vi "Measurement UI.vi"() -> ()   [LabVIEW 2021, in "audio_adc_acDualChannelMeasurementUI.lvlib"]
uses:
  audio_adc_acDualChannelMeasurementUI.lvlib
  sub-vis/View.ctl
  sub-vis/Selector.ctl
  audio_adc_acDualChannelMeasurement.lvlib
panel:
  in  "MeasGraphs":T1(tab)
  in  "freq view":T2
  out "FreqDomainGraph":cluster{"x0":dbl, "dx":dbl, "magnitude":dbl[]}[](graph) caption="AC"
  in  "time view":T2
  out "TimeDomainGraph":waveform(dbl)[](graph) caption="AC"
  in  "Bit clock edge sync":u32=1
  in  "Frame sync pulse width":u32=32
  in  "Frame length":u32=64
  in  "Data justification":u32 caption="Data Justification"
  in  "Endianness":u32
  in  "Channel 0 offset":u32=1
  in  "Bit depth":u32=24
  in  "Channel length":u32=32
  in  "Channel count per frame":u32=2
  in  "Frame sync edge for channel 0":u32=1
  out "Spectrum":dbl[](array[numeric])
  out "df":dbl[](array[numeric])
  out "f0":dbl[](array[numeric])
  out "Time domain":dbl[](array[numeric])
  out "dt":dbl[](array[numeric])
  out "THD+N":dbl[](array[numeric])
  out "THD":dbl[](array[numeric])
  out "SNR":dbl[](array[numeric])
  out "Calculated amplitude":dbl[](array[numeric])
  out "Calculated frequency":dbl[](array[numeric])
  out "SFDR":dbl[](array[numeric])
  out "Dynamic range":dbl[](array[numeric])
  out "Gain error":dbl[](array[numeric])
  out "MeasTable":string[][](table)
  in  "Select":T3
  in  "Resource List":i32[](listbox)
  in  "Analog source resource name":string caption="RESOURCE NAME"
  in  "Configure Protocol Settings":bool
  in  "Protocol capture resource name":string(combo) caption="RESOURCE NAME"
  in  "Channel":string caption="CHANNEL"
  in  "Data line":u16 caption="DATA LINE"
  in  "Protocol settings":string="Protocol settings"
  in  "Analog source":string="Analog source "
  in  "Full scale range":dbl=2.825 caption="FULL SCALE RANGE" format="%.3pV"
  in  "Measurement settings":string="Measurement settings"
  in  "MeasSettingsOptions":i32(listbox)=-1
  in  "MeasSettings":bool
  in  "Weighting filter":string(combo)="Linear" caption="WEIGHTING FILTER"
  in  "Measurement duration":dbl=0.1 caption="MEASUREMENT DURATION" format="%#_6ps"
  in  "Sample rate":dbl=44100.0 caption="SAMPLE RATE" format="%#.6pHz"
  in  "Band stop":dbl=20000.0 caption="BAND STOP" format="%#_6pHz"
  in  "Band start":dbl=20.0 caption="BAND START" format="%#_6pHz"
  in  "Amplitude":dbl=-1.0 caption="AMPLITUDE" format="%#_6pdB"
  in  "Frequency":dbl=1000.0 caption="FREQUENCY" format="%#_6pHz"
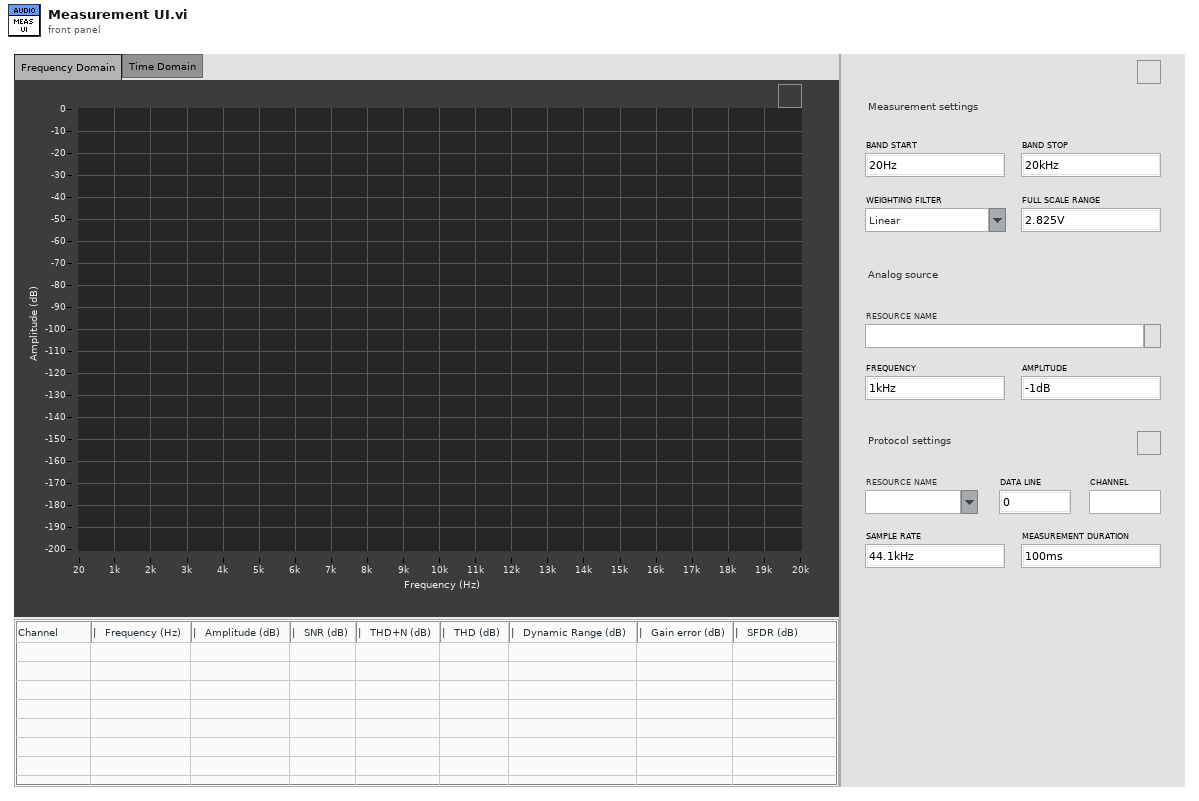
[diagram p1: front panel]
types:
  T1 = enum32{"Frequency Domain", "Time Domain", "Hidden Controls"}
  T2 = typedef "audio_adc_acDualChannelMeasurement.lvlib/View.ctl" = bool
  T3 = typedef "audio_adc_acDualChannelMeasurement.lvlib/Selector.ctl" = bool
  T4 = enum16{"open", "replace", "create", "open or create", "replace or create", "replace or create with confirmation"}
  T5 = typedef "LVRectTypeDef.ctl" = cluster{"Left":i16, "Top":i16, "Right":i16, "Bottom":i16}
  T6 = typedef "PDM Shared.lvlib/PCM Frame Sync Control.ctl" = cluster{"Frame Length":u16, "Frame Sync Pulse Width":u16, "Bit Clock Edge  Sync":T7}
  T7 = typedef "PDM Shared.lvlib/Digital Edge.ctl" = enum8{"Rising", "Falling"}
  T8 = typedef "PDM Shared.lvlib/PCM Data Format Configuration.ctl" = cluster{"Frame Sync Edge for Channel 0":T7, "Channel Count Per Frame":u8, "Channel Length":u16, "Bit Depth":u8, "Channel 0 Offset":u16, "Endianness":T9, "Data Justification":T10}
  T9 = typedef "PDM Shared.lvlib/PCM Bit Endianness.ctl" = enum16{"MSB First", "LSB First"}
  T10 = typedef "PDM Shared.lvlib/PCM Data Justification.ctl" = enum16{"Left Justified", "Right Justified"}
  T11 = typedef "LVPoint32TypeDef.ctl" = cluster{"Horizontal":i32, "Vertical":i32}
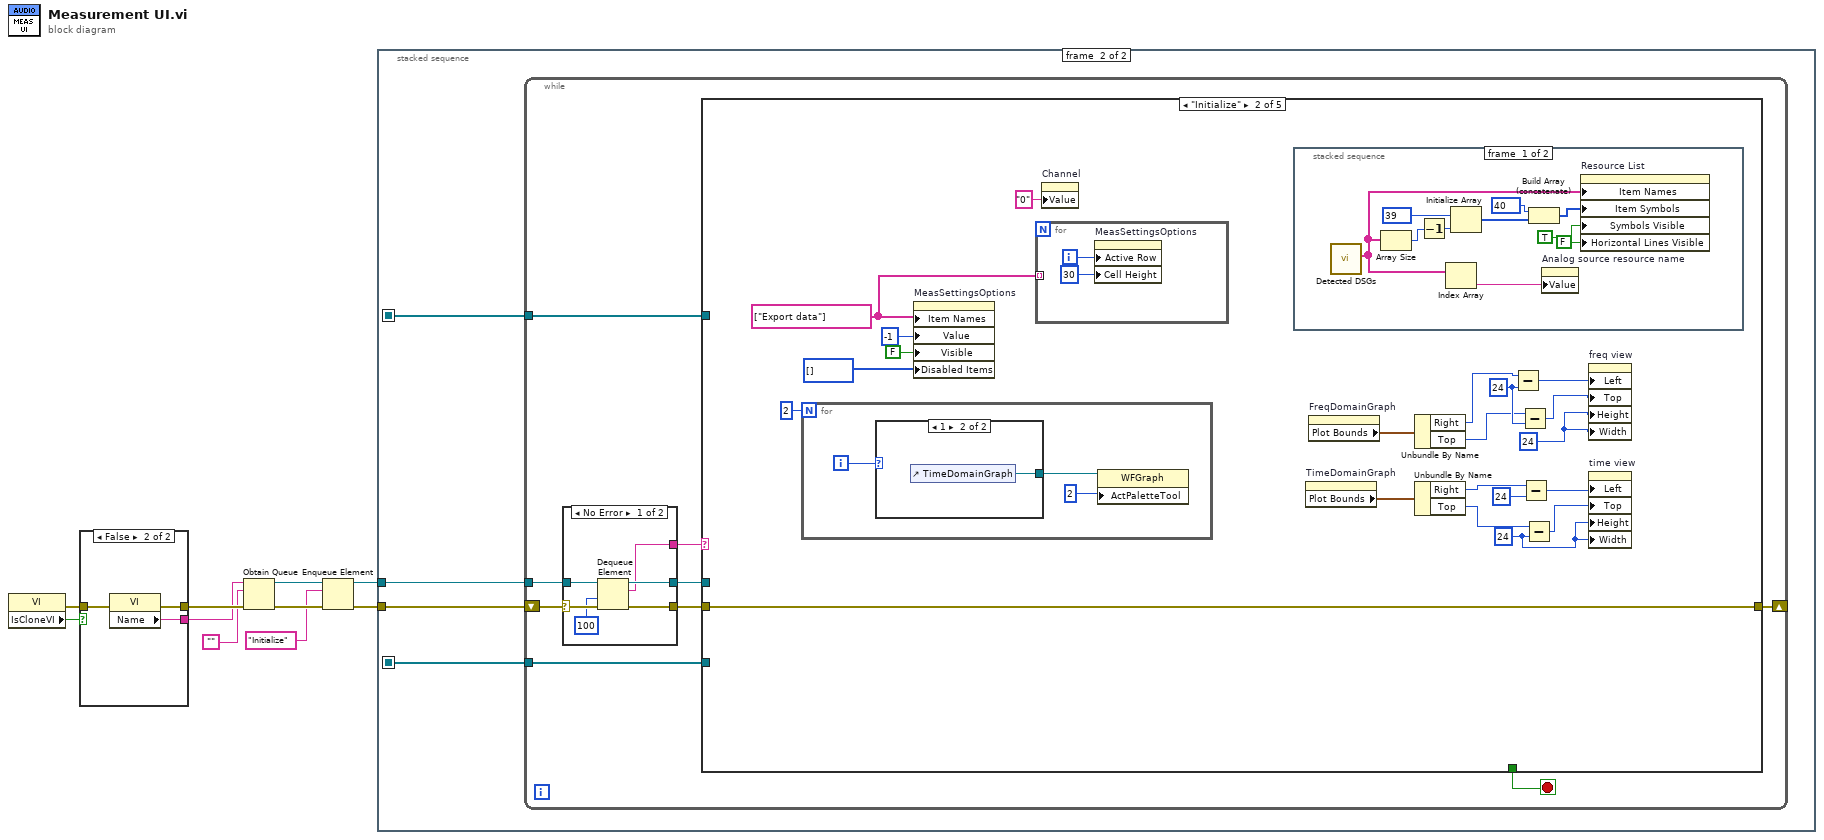
[diagram p0: block diagram]
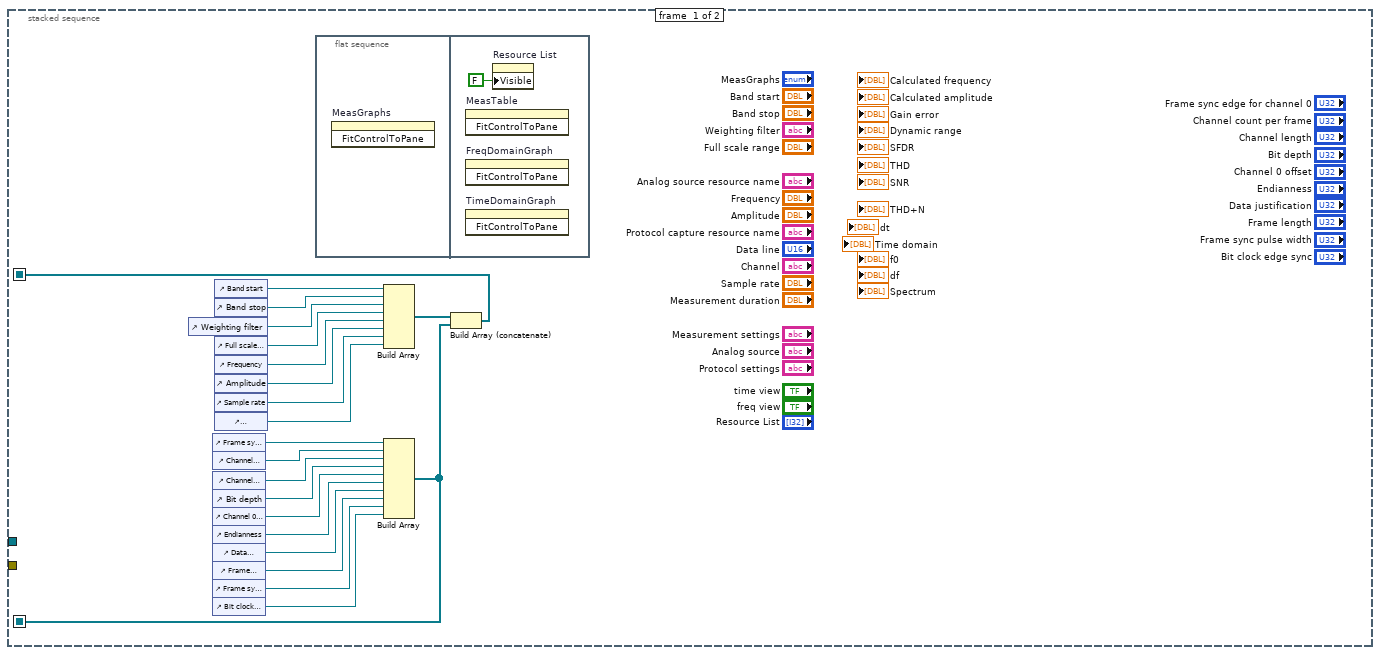
[diagram p2: hidden frame]
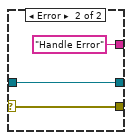
[diagram p3: hidden frame]
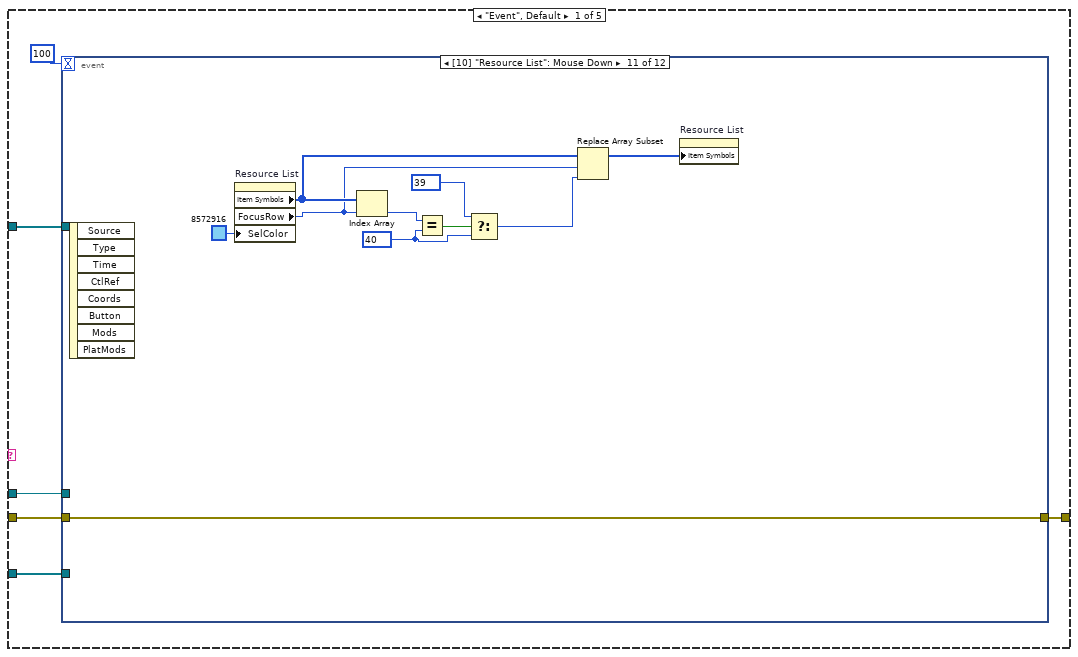
[diagram p4: hidden frame]
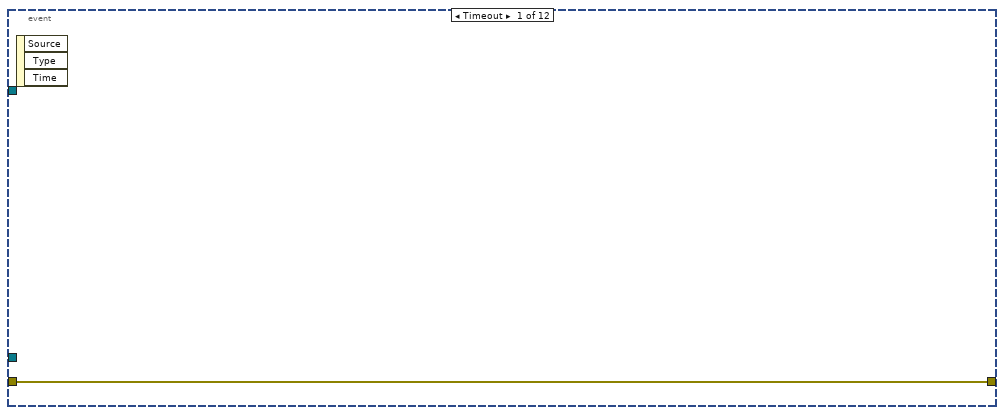
[diagram p5: hidden frame]
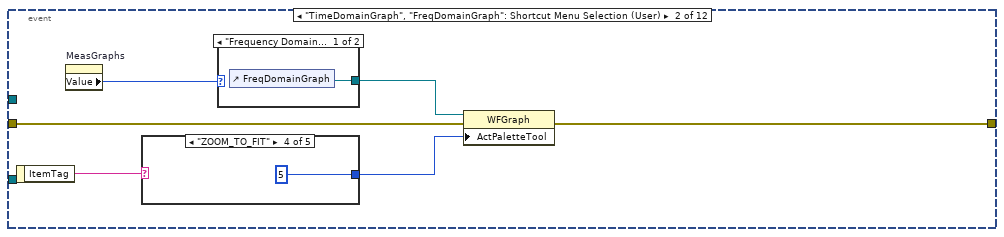
[diagram p6: hidden frame]
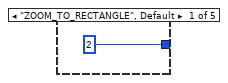
[diagram p7: hidden frame]
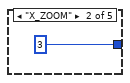
[diagram p8: hidden frame]
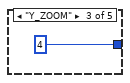
[diagram p9: hidden frame]
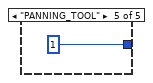
[diagram p10: hidden frame]
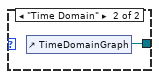
[diagram p11: hidden frame]
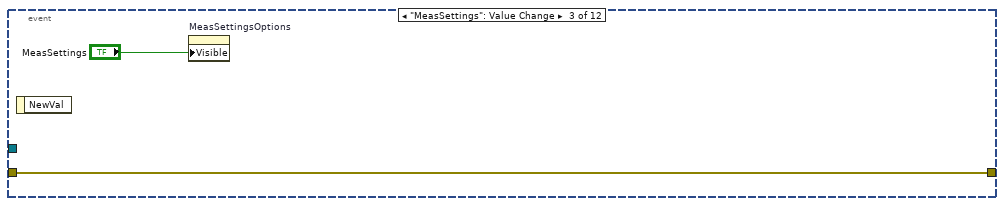
[diagram p12: hidden frame]
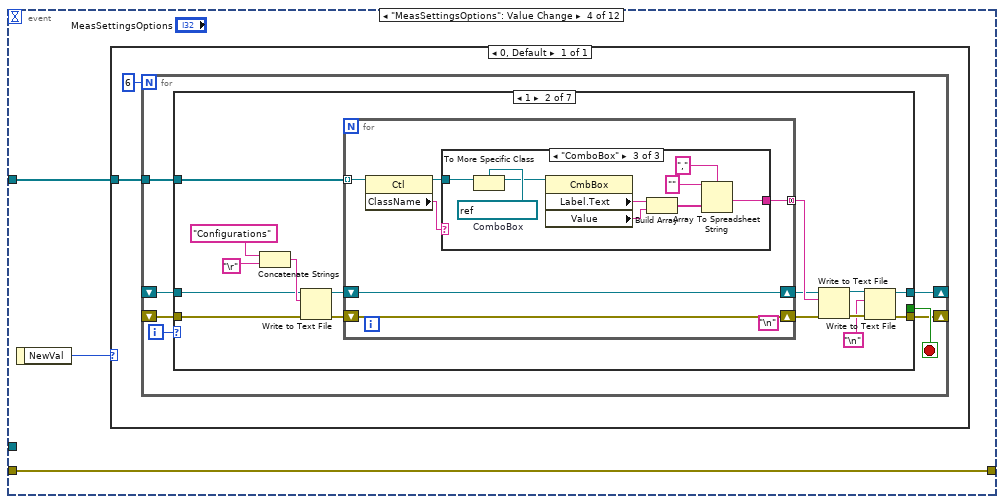
[diagram p13: hidden frame]
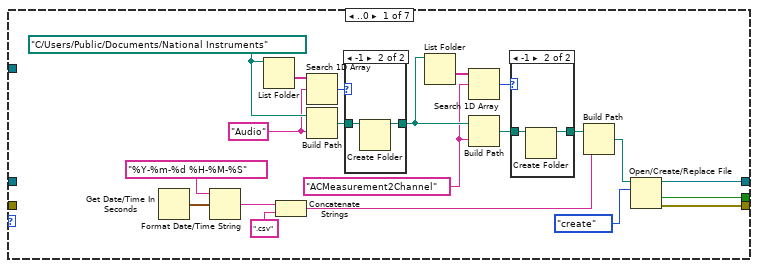
[diagram p14: hidden frame]
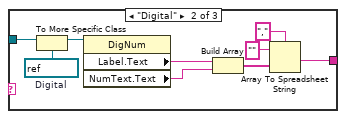
[diagram p18: hidden frame]
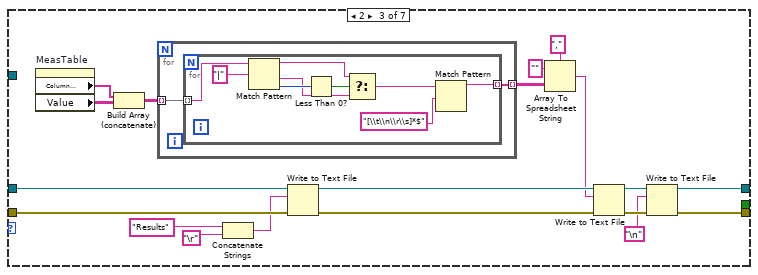
[diagram p19: hidden frame]
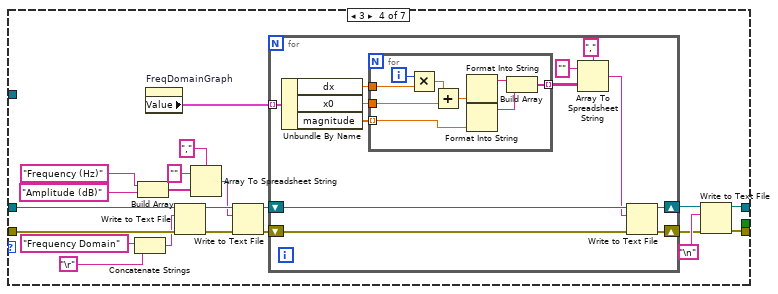
[diagram p20: hidden frame]
diagram:
  n1 = property class="VI"() -> (error out=w1:errorcluster, "IsCloneVI"=w2:bool)  [unwired: 2 in, 1 out]
  n2 = case shown="False" w2 {
    tunnel: [w13 w16] -> w10
    tunnel: [w12 w15] -> w9
    tunnel: w1 -> [w11 w14]
    frame True {
      n3 = property class="VI"(error in=w11) -> (error out=w13:errorcluster, "Clone Name"=w12:string)  [unwired: 1 in, 1 out]
    }
    frame False {
      n4 = property class="VI"(error in=w14) -> (error out=w16:errorcluster, "Name"=w15:string)  [unwired: 1 in, 1 out]
    }
  }
  n5 = Obtain Queue(name (unnamed)=w9, element data type="", error in (no error)=w10) -> (queue out=w6:refnum<queue>, error out=w8:errorcluster)  [unwired: 2 in, 1 out]
  n6 = Enqueue Element(queue=w6, element="Initialize", error in (no error)=w8) -> (queue out=w5:refnum<queue>, error out=w7:errorcluster)  [unwired: 1 in, 1 out]
  n7 = stacked-sequence {
    seq-local: [w17 _] -> [_ w40]
    seq-local: [w18 _] -> [_ w39]
    tunnel: w7 -> [_ w42]
    tunnel: w5 -> [_ w41]
    frame #0 {
      n8 = control-ref of="Weighting filter"() -> (w35:refnum<vi>)
      n9 = control-ref of="Frame sync edge for channel 0"() -> (w29:refnum<vi>)
      n10 = control-ref of="Channel count per frame"() -> (w28:refnum<vi>)
      n11 = control-ref of="Channel length"() -> (w27:refnum<vi>)
      n12 = control-ref of="Bit depth"() -> (w20:refnum<vi>)
      n13 = control-ref of="Channel 0 offset"() -> (w26:refnum<vi>)
      n14 = control-ref of="Endianness"() -> (w25:refnum<vi>)
      n15 = control-ref of="Data justification"() -> (w24:refnum<vi>)
      n16 = control-ref of="Frame length"() -> (w23:refnum<vi>)
      n17 = control-ref of="Frame sync pulse width"() -> (w22:refnum<vi>)
      n18 = control-ref of="Bit clock edge sync"() -> (w21:refnum<vi>)
      n19 = control-ref of="Band start"() -> (w37:refnum<vi>)
      n20 = control-ref of="Band stop"() -> (w36:refnum<vi>)
      n21 = control-ref of="Full scale range"() -> (w34:refnum<vi>)
      n22 = control-ref of="Frequency"() -> (w33:refnum<vi>)
      n23 = control-ref of="Amplitude"() -> (w32:refnum<vi>)
      n24 = control-ref of="Sample rate"() -> (w31:refnum<vi>)
      n25 = control-ref of="Measurement duration"() -> (w30:refnum<vi>)
      n26 = flat-sequence {
        frame #0 {
          n27 = invoke on="MeasGraphs" class="TabCtl (strict)" method="FitControlToPane"() -> ()  [unwired: 3 in, 3 out]
        }
        frame #1 {
          n28 = invoke on="MeasTable" class="Tbl (strict)" method="FitControlToPane"() -> ()  [unwired: 3 in, 3 out]
          n29 = invoke on="FreqDomainGraph" class="WFGraph (strict)" method="FitControlToPane"() -> ()  [unwired: 3 in, 3 out]
          n30 = invoke on="TimeDomainGraph" class="WFGraph (strict)" method="FitControlToPane"() -> ()  [unwired: 3 in, 3 out]
          n31 = property on="Resource List" class="LstBox (strict)"("Visible"=FALSE) -> ()  [unwired: 2 in, 2 out]
        }
      }
      n32 = Build Array(w37, w36, w35, w34, w33, w32, w31, w30) -> (w19:refnum<vi>[])
      n33 = Build Array(w29, w28, w27, w20, w26, w25, w24, w23, w22, w21) -> (w18:refnum<vi>[])
      n34 = Build Array (concatenate)(w19, w18) -> (w17:refnum<vi>[])
    }
    frame #1 {
      n35 = while {
        shift-right: [w46] -> _
        shift-left: w42 -> [w51]
        tunnel: w41 -> [w49]
        tunnel: w40 -> [w44]
        tunnel: w39 -> [w43]
        stop <- w45 stop-if-true
        n36 = case shown="No Error" w51 {
          selector: w51 -> [w57 w60]
          tunnel: [w56 w60] -> w50
          tunnel: w49 -> [w55 w59]
          tunnel: [w54 w59] -> w48
          tunnel: [w53 "Handle Error"] -> w47
          frame No Error {
            n37 = Dequeue Element(queue=w55, timeout in ms (-1)=100, error in (no error)=w57) -> (queue out=w54:refnum<queue>, element=w53:string, error out=w56:errorcluster)  [unwired: 1 out]
          }
          frame Error {
          }
        }
        n38 = case shown="\"Initialize\"" w47 {
          tunnel: w50 -> [w65 w406 w460 w530 w531]
          tunnel: w48 -> [w63 _ _ w528 _]
          tunnel: [w66 w406 w460 w525 w531] -> w46
          tunnel: [_ _ _ TRUE _] -> w45
          tunnel: w44 -> [w62 _ _ _ _]
          tunnel: w43 -> [w61 _ _ _ _]
          frame "Event", Default {
            n39 = event shown="[10] \"Resource List\": Mouse Down" {
              selector: _ -> [_ _ _ _ _ _ _ _ _ _ _ _]
              dyn-events: _ -> [_ _ _ _ _ _ _ _ _ _ _ _]
              timeout: 100 -> [_ _ _ _ _ _ _ _ _ _ _ _]
              tunnel: [w67 w70 _ w85 w278 _ _ _ w331 w353 w371 w383] -> w66
              tunnel: w65 -> [w67 w69 w81 w85 w278 _ _ _ w331 w353 w371 w384]
              tunnel: w63 -> [_ _ _ _ _ _ _ _ _ _ _ w382]
              tunnel: [_ _ w81 _ _ _ _ _ _ _ _ _] -> _
              tunnel: w62 -> [_ _ _ w83 _ _ _ _ _ _ _ _]
              tunnel: w61 -> [_ _ _ _ _ _ _ w311 _ _ _ _]
              event Timeout {
                n40 = event-data() -> ()  [unwired: 1 in, 3 out]
              }
              event "TimeDomainGraph", "FreqDomainGraph": Shortcut Menu Selection (User) {
                n41 = event-data() -> ("ItemTag"=w72:string)  [unwired: 1 in]
                n42 = property on="MeasGraphs" class="TabCtl (strict)"() -> ("Value"=w73:T1)  [unwired: 2 in, 2 out]
                n43 = case shown="\"ZOOM_TO_FIT\"" w72 {
                  tunnel: [2 3 4 5 1] -> w68
                  frame "ZOOM_TO_RECTANGLE", Default {
                  }
                  frame "X_ZOOM" {
                  }
                  frame "Y_ZOOM" {
                  }
                  frame "ZOOM_TO_FIT" {
                  }
                  frame "PANNING_TOOL" {
                  }
                }
                n44 = case shown="\"Frequency Domain\", Default" w73 {
                  tunnel: [w79 w80] -> w71
                  frame "Frequency Domain", Default {
                    n45 = control-ref of="FreqDomainGraph"() -> (w79:refnum<vi>)
                  }
                  frame "Time Domain" {
                    n46 = control-ref of="TimeDomainGraph"() -> (w80:refnum<vi>)
                  }
                }
                n47 = property class="WFGraph"(reference=w71, error in=w69, "ActPaletteTool"=w68) -> (error out=w70:errorcluster)  [unwired: 1 out]
              }
              event "MeasSettings": Value Change {
                n48 = event-data() -> ()  [unwired: 1 in, 1 out]
                n49 = property on="MeasSettingsOptions" class="LstBox (strict)"("Visible"="MeasSettings") -> ()  [unwired: 2 in, 2 out]
              }
              event "MeasSettingsOptions": Value Change {
                n50 = event-data() -> ("NewVal"=w84:i32)  [unwired: 1 in]
                n51 = case shown="0, Default" w84 {
                  tunnel: w83 -> [w86]
                  frame 0, Default {
                    n52 = for {
                      N: 6 -> [_]
                      shift-right: [w92] -> _
                      shift-left: _ -> [w91]
                      shift-right: [w90] -> _
                      shift-left: _ -> [w89]
                      tunnel: w86 -> [w88]
                      i -> [w94]
                      stop <- w93 stop-if-true
                      n53 = case shown="1" w94 {
                        tunnel: [w108 _ _ _ _ _ _] -> w93
                        tunnel: [w114 w134 w169 w194 w240 refnum<file> refnum ("refnum out") w277] -> w92
                        tunnel: w91 -> [_ w131 w180 w212 w241 w275 w277]
                        tunnel: [w107 w133 w168 w192 w239 w273 w276] -> w90
                        tunnel: w89 -> [_ w129 w179 w211 w242 w272 w276]
                        tunnel: w88 -> [_ w132 _ _ _ _ _]
                        frame ..0 {
                          w103 = "ACMeasurement2Channel" ("prompt")
                          w110 = "Audio" ("prompt")
                          w113 = path "C:/Users/Public/Documents/National Instruments" ("base path")
                          n54 = Get Date/Time In Seconds() -> (seconds since 1Jan1904=w100:timestamp)
                          n55 = Format Date/Time String(time format string (%c)="%Y-%m-%d %H-%M-%S", seconds (now)=w100) -> (date/time string=w99:string)  [unwired: 1 in]
                          n56 = List Folder(path=w113) -> (folder names=w111:string[])  [unwired: 3 in, 3 out]
                          n57 = Concatenate Strings(w99, ".csv" ("string")) -> (w96:string)
                          n58 = Search 1D Array(1D array=w111, element=w110) -> (index of element=w109:i32)  [unwired: 1 in]
                          n59 = Build Path(base path=w113, name or relative path=w110) -> (appended path=w112:path)
                          n60 = case shown="-1" w109 {
                            tunnel: w112 -> [w119 w121]
                            tunnel: [w119 w120] -> w104
                            frame Default {
                            }
                            frame -1 {
                              n61 = Create Folder(path (use dialog)=w121) -> (created path=w120:path)  [unwired: 2 in, 2 out]
                            }
                          }
                          n62 = List Folder(path=w104) -> (folder names=w106:string[])  [unwired: 3 in, 3 out]
                          n63 = Search 1D Array(1D array=w106, element=w103) -> (index of element=w105:i32)  [unwired: 1 in]
                          n64 = Build Path(base path=w104, name or relative path=w103) -> (appended path=w102:path)
                          n65 = case shown="-1" w105 {
                            tunnel: w102 -> [w116 w118]
                            tunnel: [w116 w117] -> w97
                            frame Default {
                            }
                            frame -1 {
                              n66 = Create Folder(path (use dialog)=w118) -> (created path=w117:path)  [unwired: 2 in, 2 out]
                            }
                          }
                          n67 = Build Path(base path=w97, name or relative path=w96) -> (appended path=w95:path)
                          n68 = Open/Create/Replace File(file path (use dialog)=w95, operation (0:open)=T4."create") -> (refnum out=w114:refnum<file>, cancelled=w108:bool, error out=w107:errorcluster)  [unwired: 4 in]
                        }
                        frame 1 {
                          (unwired) "\n"
                          n69 = Concatenate Strings("Configurations" ("format string"), "\r") -> (w135:string)
                          n70 = Write to Text File(file (use dialog)=w131, text=w135, error in=w129) -> (refnum out=w128:refnum<file>, error out=w130:errorcluster)  [unwired: 1 in, 1 out]
                          n71 = for {
                            tunnel: w132 -> [w139] mode=indexing
                            shift-right: [w143] -> w126
                            shift-left: w128 -> [w143]
                            shift-right: [w142] -> w125
                            shift-left: w130 -> [w142]
                            tunnel: [w141] -> w127 mode=concatenating
                            n72 = property class="Ctl"(reference=w139) -> (reference out=w140:refnum<vi>, "ClassName"=w138:string)  [unwired: 1 in, 1 out]
                            n73 = case shown="\"ComboBox\"" w138 {
                              tunnel: [_ w147 w157] -> w141
                              tunnel: w140 -> [_ w145 w161]
                              frame Default {
                              }
                              frame "Digital" {
                                w144 = refnum<vi> refnum  # Digital
                                n74 = To More Specific Class(target class=w144, reference=w145) -> (specific class reference=w146:refnum<vi>)  [unwired: 1 in, 1 out]
                                n75 = property class="DigNum"(reference=w146) -> ("Label.Text"=w152:string, "NumText.Text"=w151:string)  [unwired: 1 in, 2 out]
                                n76 = Build Array(w152, w151) -> (w148:string[])
                                n77 = Array To Spreadsheet String(delimiter (Tab)=",", array=w148, 3:"" ("format string")) -> (spreadsheet string=w147:string)
                              }
                              frame "ComboBox" {
                                w160 = refnum<vi> refnum  # ComboBox
                                n78 = To More Specific Class(target class=w160, reference=w161) -> (specific class reference=w156:refnum<vi>)  [unwired: 1 in, 1 out]
                                n79 = property class="CmbBox"(reference=w156) -> ("Label.Text"=w155:string, "Value"=w154:string)  [unwired: 1 in, 2 out]
                                n80 = Build Array(w155, w154) -> (w153:string[])
                                n81 = Array To Spreadsheet String(delimiter (Tab)=",", array=w153, 3:"" ("format string")) -> (spreadsheet string=w157:string)
                              }
                            }
                          }
                          n82 = Write to Text File(file (use dialog)=w126, text=w127, error in=w125) -> (refnum out=w124:refnum<file>, error out=w123:errorcluster)  [unwired: 1 in, 1 out]
                          n83 = Write to Text File(file (use dialog)=w124, text="\n", error in=w123) -> (refnum out=w134:refnum<file>, error out=w133:errorcluster)  [unwired: 1 in, 1 out]
                        }
                        frame 2 {
                          n84 = property on="MeasTable" class="Tbl (strict)"() -> ("Column Headers[]"=w163:string[], "Value"=w162:string[][])  [unwired: 2 in, 2 out]
                          n85 = Build Array (concatenate)(w163, w162) -> (w177:string[][])
                          n86 = for {
                            tunnel: w177 -> [w182] mode=indexing
                            tunnel: [w181] -> w176 mode=indexing
                            n87 = for {
                              tunnel: w182 -> [w184] mode=indexing
                              tunnel: [w183] -> w181 mode=indexing
                              n88 = Match Pattern(string=w184, regular expression="|") -> (before substring=w188:string, after substring=w187:string, offset past match=w190:i32)  [unwired: 1 in, 1 out]
                              n89 = Less Than 0?(x=w190) -> (x < 0?=w189:bool)
                              n90 = Select(t=w188, s=w189, f=w187) -> (s? t:f=w186:string)
                              n91 = Match Pattern(string=w186, regular expression="[\\t\\n\\r\\s]*$") -> (before substring=w183:string)  [unwired: 1 in, 3 out]
                            }
                          }
                          n92 = Concatenate Strings("Results" ("element"), "\r") -> (w164:string)
                          n93 = Write to Text File(file (use dialog)=w180, text=w164, error in=w179) -> (refnum out=w178:refnum<file>, error out=w172:errorcluster)  [unwired: 1 in, 1 out]
                          n94 = Array To Spreadsheet String(delimiter (Tab)=",", array=w176, 3:"" ("format string")) -> (spreadsheet string=w173:string)
                          n95 = Write to Text File(file (use dialog)=w178, text=w173, error in=w172) -> (refnum out=w171:refnum<file>, error out=w170:errorcluster)  [unwired: 1 in, 1 out]
                          n96 = Write to Text File(file (use dialog)=w171, text="\n", error in=w170) -> (refnum out=w169:refnum<file>, error out=w168:errorcluster)  [unwired: 1 in, 1 out]
                        }
                        frame 3 {
                          n97 = Concatenate Strings("Frequency Domain" ("string"), "\r") -> (w209:string)
                          n98 = Build Array("Frequency (Hz)", "Amplitude (dB)") -> (w208:string[])
                          n99 = property on="FreqDomainGraph" class="WFGraph (strict)"() -> ("Value"=w199:cluster{"x0":dbl, "dx":dbl, "magnitude":dbl[]}[])  [unwired: 2 in, 2 out]
                          n100 = Write to Text File(file (use dialog)=w212, text=w209, error in=w211) -> (refnum out=w205:refnum<file>, error out=w204:errorcluster)  [unwired: 1 in, 1 out]
                          n101 = Array To Spreadsheet String(delimiter (Tab)=",", array=w208, 3:"" ("format string")) -> (spreadsheet string=w203:string)
                          n102 = Write to Text File(file (use dialog)=w205, text=w203, error in=w204) -> (refnum out=w202:refnum<file>, error out=w201:errorcluster)  [unwired: 1 in, 1 out]
                          n103 = for {
                            tunnel: w199 -> [w215] mode=indexing
                            shift-right: [w214] -> w195
                            shift-left: w202 -> [w224]
                            shift-right: [w213] -> w193
                            shift-left: w201 -> [w223]
                            n104 = Unbundle By Name(w215) -> ("dx"=w218:dbl, "x0"=w219:dbl, "magnitude"=w217:dbl[])
                            n105 = for {
                              tunnel: w217 -> [w228] mode=indexing
                              tunnel: w218 -> [w232]
                              tunnel: w219 -> [w230]
                              tunnel: [w225] -> w220 mode=indexing
                              i -> [w233]
                              n106 = Multiply(x=w233, y=w232) -> (x*y=w231:dbl)
                              n107 = Add(x=w231, y=w230) -> (x+y=w229:dbl)
                              n108 = Format Into String(w229) -> (resulting string=w226:string)  [unwired: 3 in, 1 out]
                              n109 = Format Into String(w228) -> (resulting string=w227:string)  [unwired: 3 in, 1 out]
                              n110 = Build Array(w226, w227) -> (w225:string[])
                            }
                            n111 = Array To Spreadsheet String(delimiter (Tab)=",", array=w220, 3:"" ("format string")) -> (spreadsheet string=w216:string)
                            n112 = Write to Text File(file (use dialog)=w224, text=w216, error in=w223) -> (refnum out=w214:refnum<file>, error out=w213:errorcluster)  [unwired: 1 in, 1 out]
                          }
                          n113 = Write to Text File(file (use dialog)=w195, text="\n", error in=w193) -> (refnum out=w194:refnum<file>, error out=w192:errorcluster)  [unwired: 1 in, 1 out]
                        }
                        frame 4 {
                          n114 = Concatenate Strings("Time Domain" ("string"), "\r") -> (w250:string)
                          n115 = Write to Text File(file (use dialog)=w241, text=w250, error in=w242) -> (refnum out=w247:refnum<file>, error out=w246:errorcluster)  [unwired: 1 in, 1 out]
                          n116 = Build Array("Time (s)", "Amplitude (V)") -> (w249:string[])
                          n117 = property on="TimeDomainGraph" class="WFGraph (strict)"() -> ("Value"=w238:waveform(dbl)[])  [unwired: 2 in, 2 out]
                          n118 = Array To Spreadsheet String(delimiter (Tab)=",", array=w249, 3:"" ("format string")) -> (spreadsheet string=w245:string)
                          n119 = Write to Text File(file (use dialog)=w247, text=w245, error in=w246) -> (refnum out=w244:refnum<file>, error out=w243:errorcluster)  [unwired: 1 in, 1 out]
                          n120 = for {
                            tunnel: w238 -> [w254] mode=indexing
                            shift-right: [w256] -> w240
                            shift-left: w244 -> [w262]
                            shift-right: [w255] -> w239
                            shift-left: w243 -> [w261]
                            n121 = Unbundle By Name(w254) -> ("dt"=w252:dbl, "Y"=w253:dbl[])
                            n122 = for {
                              tunnel: [w267] -> w258 mode=indexing
                              tunnel: w253 -> [w266] mode=indexing
                              tunnel: w252 -> [w264]
                              i -> [w265]
                              n123 = Multiply(x=w264, y=w265) -> (x*y=w263:dbl)
                              n124 = Format Into String(w263) -> (resulting string=w268:string)  [unwired: 3 in, 1 out]
                              n125 = Format Into String(w266) -> (resulting string=w269:string)  [unwired: 3 in, 1 out]
                              n126 = Build Array(w268, w269) -> (w267:string[])
                            }
                            n127 = Array To Spreadsheet String(delimiter (Tab)=",", array=w258, 3:"" ("format string")) -> (spreadsheet string=w257:string)
                            n128 = Write to Text File(file (use dialog)=w262, text=w257, error in=w261) -> (refnum out=w256:refnum<file>, error out=w255:errorcluster)  [unwired: 1 in, 1 out]
                          }
                        }
                        frame 5 {
                          w270 = FALSE ("Visible")
                          n129 = Close File(refnum=w275, error in=w272) -> (error out=w273:errorcluster)  [unwired: 1 out]
                          n130 = property on="MeasSettingsOptions" class="LstBox (strict)"("Visible"=w270, "Value"=-1 ("MeasSettingsOptions")) -> ()  [unwired: 2 in, 2 out]
                          n131 = property on="MeasSettings" class="Bool (strict)"("Value"=w270) -> ()  [unwired: 2 in, 2 out]
                        }
                        frame Default {
                        }
                      }
                    }
                  }
                }
              }
              event Pane Size {
                w279 = i16 24 ("y")
                w280 = 24
                w292 = 24
                n132 = event-data() -> ()  [unwired: 1 in, 6 out]
                n133 = flat-sequence {
                  frame #0 {
                    n134 = invoke on="MeasGraphs" class="TabCtl (strict)" method="FitControlToPane"() -> ()  [unwired: 3 in, 3 out]
                  }
                  frame #1 {
                    n135 = invoke on="FreqDomainGraph" class="WFGraph (strict)" method="FitControlToPane"() -> ()  [unwired: 3 in, 3 out]
                    n136 = invoke on="TimeDomainGraph" class="WFGraph (strict)" method="FitControlToPane"() -> ()  [unwired: 3 in, 3 out]
                    n137 = invoke on="MeasTable" class="Tbl (strict)" method="FitControlToPane"() -> ()  [unwired: 3 in, 3 out]
                  }
                }
                n138 = property on="TimeDomainGraph" class="WFGraph (strict)"() -> ("Plot Bounds"=w285:T5)  [unwired: 2 in, 2 out]
                n139 = property on="FreqDomainGraph" class="WFGraph (strict)"() -> ("Plot Bounds"=w286:T5)  [unwired: 2 in, 2 out]
                n140 = Unbundle By Name(w286) -> ("Right"=w291:i16, "Top"=w290:i16)
                n141 = Unbundle By Name(w285) -> ("Right"=w289:i16, "Top"=w287:i16)
                n142 = Subtract(x=w291, y=w292) -> (x-y=w284:i32)
                n143 = Subtract(x=w290, y=w292) -> (x-y=w283:i32)
                n144 = Subtract(x=w289, y=24) -> (x-y=w282:i32)
                n145 = Subtract(x=w287, y=w279) -> (x-y=w281:i16)
                n146 = property on="freq view" class="Bool"("Left"=w284, "Top"=w283, "Height"=w280, "Width"=w280) -> ()  [unwired: 2 in, 2 out]
                n147 = property on="time view" class="Bool"("Left"=w282, "Top"=w281, "Height"=w279, "Width"=w279) -> ()  [unwired: 2 in, 2 out]
              }
              event Value Change {
                n148 = event-data() -> ("NewVal"=w293:T2)  [unwired: 1 in]
                n149 = flat-sequence {
                  tunnel: w293 -> [w294]
                  frame #0 {
                    n150 = property on="FreqDomainGraph" class="WFGraph (strict)"("Legend Visible"=w294) -> ()  [unwired: 2 in, 2 out]
                  }
                  frame #1 {
                    n151 = property on="freq view" class="Bool"() -> ("Left"=w301:i32, "Width"=w300:u32, "Top"=w297:i32, "Height"=w296:u32)  [unwired: 2 in, 2 out]
                    n152 = property on="FreqDomainGraph" class="WFGraph (strict)"() -> ("LegWidth"=w299:u32)  [unwired: 2 in, 2 out]
                    n153 = Add(x=w297, y=w296) -> (x+y=w295:u32)
                    n154 = Compound Arithmetic op=ADD(w301, w300, invert w299) -> (w298:u32)
                    n155 = property on="FreqDomainGraph" class="WFGraph (strict)"("LegLeft"=w298, "LegTop"=w295) -> ()  [unwired: 2 in, 2 out]
                  }
                }
              }
              event Value Change {
                n156 = event-data() -> ("NewVal"=w302:T2)  [unwired: 1 in]
                n157 = flat-sequence {
                  tunnel: w302 -> [w303]
                  frame #0 {
                    n158 = property on="TimeDomainGraph" class="WFGraph (strict)"("Legend Visible"=w303) -> ()  [unwired: 2 in, 2 out]
                  }
                  frame #1 {
                    n159 = property on="time view" class="Bool"() -> ("Left"=w310:i32, "Width"=w309:u32, "Top"=w306:i32, "Height"=w305:u32)  [unwired: 2 in, 2 out]
                    n160 = property on="TimeDomainGraph" class="WFGraph (strict)"() -> ("LegWidth"=w308:u32)  [unwired: 2 in, 2 out]
                    n161 = Add(x=w306, y=w305) -> (x+y=w304:u32)
                    n162 = Compound Arithmetic op=ADD(w310, w309, invert w308) -> (w307:u32)
                    n163 = property on="TimeDomainGraph" class="WFGraph (strict)"("LegLeft"=w307, "LegTop"=w304) -> ()  [unwired: 2 in, 2 out]
                  }
                }
              }
              event "Configure Protocol Settings": Value Change {
                n164 = event-data() -> ()  [unwired: 1 in, 1 out]
                n165 = call "Protocol Settings.vi"() -> ("Frame sync clock control"=w313:T6, "PDM data configuration"=w312:T8)  [unwired: 10 in]
                n166 = call "Update Protocol UI Controls.vi"("Frame Sync Clock Control"=w313, "PCM Data Configuration"=w312, "Control references"=w311) -> ()  [unwired: 9 in]
              }
              event Mouse Down {
                w332 = FALSE ("Visible")
                n167 = event-data() -> ("Coords"=w330:T11)  [unwired: 1 in, 4 out]
                n168 = Unbundle By Name(w330) -> ("Horizontal"=w327:i32, "Vertical"=w326:i32)
                n169 = property on="Resource List" class="LstBox (strict)"() -> ("Visible"=w318:bool, "Left"=w322:i32, "Width"=w329:u32, "Top"=w323:i32, "Height"=w328:u32)  [unwired: 2 in, 2 out]
                n170 = Add(x=w323, y=w328) -> (x+y=w324:u32)
                n171 = property on="MeasSettingsOptions" class="LstBox (strict)"("Visible"=w332, "Value"=-1 ("MeasSettingsOptions")) -> ()  [unwired: 2 in, 2 out]
                n172 = Add(x=w322, y=w329) -> (x+y=w325:u32)
                n173 = In Range and Coerce(upper limit=w325, x=w327, lower limit=w322) -> (In Range?=w321:bool)  [unwired: 1 out]
                n174 = In Range and Coerce(upper limit=w324, x=w326, lower limit=w323) -> (In Range?=w320:bool)  [unwired: 1 out]
                n175 = And(x=w321, y=w320) -> (x .and. y?=w319:bool)
                n176 = Equal?(x=w318, y=TRUE) -> (x = y?=w316:bool)
                n177 = Not(x=w319) -> (.not. x?=w315:bool)
                n178 = property on="MeasSettings" class="Bool (strict)"("Value"=w332) -> ()  [unwired: 2 in, 2 out]
                n179 = And(x=w316, y=w315) -> (x .and. y?=w314:bool)
                n180 = case shown="True" w314 {
                  frame False {
                  }
                  frame True {
                    n181 = property on="Resource List" class="LstBox (strict)"("Visible"=FALSE) -> ("Item Symbols"=w340:i32[], "Item Names"=w341:string[])  [unwired: 2 in, 2 out]
                    n182 = for {
                      tunnel: w341 -> [w347] mode=indexing
                      tunnel: w340 -> [w349] mode=indexing
                      tunnel: [w347] -> w339 mode=indexing if=w346
                      n183 = Equal?(x=40, y=w349) -> (x = y?=w346:bool)
                    }
                    n184 = for {
                      tunnel: w339 -> [w345] mode=indexing
                      tunnel: [w343] -> w338 mode=concatenating
                      n185 = Concatenate Strings(w345, "," ("string")) -> (w343:string)
                    }
                    n186 = String Length(string=w338) -> (length=w337:i32)
                    n187 = Decrement(x=w337) -> (x-1=w336:i32)
                    n188 = String Subset(string=w338, offset (0)=0, length (rest)=w336) -> (substring=w334:string)
                    n189 = property on="Analog source resource name" class="Str"("Value"=w334) -> ()  [unwired: 2 in, 2 out]
                  }
                }
              }
              event Value Change {
                n190 = event-data() -> ()  [unwired: 1 in, 6 out]
                n191 = property on="Resource List" class="LstBox (strict)"() -> ("Visible"=w352:bool)  [unwired: 2 in, 2 out]
                n192 = Equal?(x=w352, y=TRUE) -> (x = y?=w350:bool)
                n193 = case shown="True" w350 {
                  frame False {
                    n194 = property on="Resource List" class="LstBox (strict)"("Visible"=TRUE) -> ()  [unwired: 2 in, 2 out]
                  }
                  frame True {
                    n195 = property on="Resource List" class="LstBox (strict)"("Visible"=FALSE) -> ("Item Symbols"=w361:i32[], "Item Names"=w362:string[])  [unwired: 2 in, 2 out]
                    n196 = for {
                      tunnel: w362 -> [w368] mode=indexing
                      tunnel: w361 -> [w370] mode=indexing
                      tunnel: [w368] -> w360 mode=indexing if=w367
                      n197 = Equal?(x=40, y=w370) -> (x = y?=w367:bool)
                    }
                    n198 = for {
                      tunnel: w360 -> [w366] mode=indexing
                      tunnel: [w364] -> w359 mode=concatenating
                      n199 = Concatenate Strings(w366, "," ("string")) -> (w364:string)
                    }
                    n200 = String Length(string=w359) -> (length=w358:i32)
                    n201 = Decrement(x=w358) -> (x-1=w357:i32)
                    n202 = String Subset(string=w359, offset (0)=0, length (rest)=w357) -> (substring=w355:string)
                    n203 = property on="Analog source resource name" class="Str"("Value"=w355) -> ()  [unwired: 2 in, 2 out]
                  }
                }
              }
              event "Resource List": Mouse Down {
                w376 = 40
                n204 = event-data() -> ()  [unwired: 1 in, 8 out]
                n205 = property on="Resource List" class="LstBox (strict)"("SelColor"=u32 8572916 ("Selection Color")) -> ("Item Symbols"=w375:i32[], "FocusRow"=w374:i32)  [unwired: 2 in, 2 out]
                n206 = Index Array(array=w375, index=w374) -> (element=w379:i32)
                n207 = Equal?(x=w379, y=w376) -> (x = y?=w378:bool)
                n208 = Select(t=39, s=w378, f=w376) -> (s? t:f=w373:i32)
                n209 = Replace Array Subset(array=w375, new element=w373, index=w374) -> (w372:i32[])
                n210 = property on="Resource List" class="LstBox (strict)"("Item Symbols"=w372) -> ()  [unwired: 2 in, 2 out]
              }
              event Panel Close? {
                n211 = event-data() -> ()  [unwired: 1 in, 4 out]
                n212 = Enqueue Element(queue=w382, element="Exit", error in (no error)=w384) -> (error out=w383:errorcluster)  [unwired: 1 in, 2 out]
                n213 = event-data("Discard?"=TRUE) -> ()  [unwired: 1 in, 1 out]
              }
            }
          }
          frame "Initialize" {
            w387 = i16 24 ("y")
            w388 = 24
            w400 = 24
            w404 = string[] ["Export data"] ("Item Names")
            n214 = for {
              N: 2 -> [_]
              i -> [w422]
              n215 = case shown="1" w422 {
                tunnel: [w425 w426] -> w423
                frame 0, Default {
                  n216 = control-ref of="FreqDomainGraph"() -> (w425:refnum<vi>)
                }
                frame 1 {
                  n217 = control-ref of="TimeDomainGraph"() -> (w426:refnum<vi>)
                }
              }
              n218 = property class="WFGraph"(reference=w423, "ActPaletteTool"=2 ("Palette:Active Tool")) -> ()  [unwired: 1 in, 2 out]
            }
            n219 = property on="MeasSettingsOptions" class="LstBox (strict)"("Item Names"=w404, "Value"=-1 ("MeasSettingsOptions"), "Visible"=FALSE, "Disabled Items"=i32[] []) -> ()  [unwired: 2 in, 2 out]
            n220 = for {
              tunnel: w404 -> [_] mode=indexing
              i -> [w421]
              n221 = property on="MeasSettingsOptions" class="LstBox (strict)"("Active Row"=w421, "Cell Height"=30 ("Active Row:Cell Height")) -> ()  [unwired: 2 in, 2 out]
            }
            n222 = property on="Channel" class="Str"("Value"="0" ("Channel")) -> ()  [unwired: 2 in, 2 out]
            n223 = stacked-sequence {
              frame #0 {
                n224 = call "Detected DSGs.vi"() -> ("AO channels"=w408:string[])  [unwired: 11 in]
                n225 = Array Size(array=w408) -> (size(s)=w414:i32)
                n226 = Decrement(x=w414) -> (x-1=w413:i32)
                n227 = Index Array(array=w408) -> (element=w416:string)  [unwired: 1 in]
                n228 = Initialize Array(39, w413) -> (w411:i32[])
                n229 = Build Array (concatenate)(40, w411) -> (w410:i32[])
                n230 = property on="Analog source resource name" class="Str"("Value"=w416) -> ()  [unwired: 2 in, 2 out]
                n231 = property on="Resource List" class="LstBox (strict)"("Item Names"=w408, "Item Symbols"=w410, "Symbols Visible"=TRUE ("Visible Items:Symbols Visible"), "Horizontal Lines Visible"=FALSE ("Visible Items:Horizontal Lines Visible")) -> ()  [unwired: 2 in, 2 out]
              }
              frame #1 {
                n232 = call "Detected PDMs.vi"() -> ("PDM devices"=w419:string[])  [unwired: 11 in]
                n233 = Index Array(array=w419, index=0) -> (element=w418:string)
                n234 = property on="Protocol capture resource name" class="CmbBox"("Strings[]"=w419, "Value"=w418) -> ()  [unwired: 2 in, 2 out]
              }
            }
            n235 = property on="TimeDomainGraph" class="WFGraph (strict)"() -> ("Plot Bounds"=w393:T5)  [unwired: 2 in, 2 out]
            n236 = property on="FreqDomainGraph" class="WFGraph (strict)"() -> ("Plot Bounds"=w394:T5)  [unwired: 2 in, 2 out]
            n237 = Unbundle By Name(w394) -> ("Right"=w399:i16, "Top"=w398:i16)
            n238 = Unbundle By Name(w393) -> ("Right"=w397:i16, "Top"=w395:i16)
            n239 = Subtract(x=w399, y=w400) -> (x-y=w392:i32)
            n240 = Subtract(x=w398, y=w400) -> (x-y=w391:i32)
            n241 = Subtract(x=w397, y=24) -> (x-y=w390:i32)
            n242 = Subtract(x=w395, y=w387) -> (x-y=w389:i16)
            n243 = property on="freq view" class="Bool"("Left"=w392, "Top"=w391, "Height"=w388, "Width"=w388) -> ()  [unwired: 2 in, 2 out]
            n244 = property on="time view" class="Bool"("Left"=w390, "Top"=w389, "Height"=w387, "Width"=w387) -> ()  [unwired: 2 in, 2 out]
          }
          frame "Post UI Update" {
            w430 = 2
            # "This case will be triggered, after framework updates the User interface with result values."
            n245 = local read "Time domain"() -> (w438:dbl[])
            n246 = local read "Spectrum"() -> (w443:dbl[])
            n247 = local read "Calculated frequency"() -> (w456:dbl[])
            n248 = local read "Calculated amplitude"() -> (w455:dbl[])
            n249 = local read "dt"() -> (w437:dbl[])
            n250 = local read "df"() -> (w444:dbl[])
            n251 = local read "Dynamic range"() -> (w457:dbl[])
            n252 = property on="Channel" class="Str"() -> ("Value"=w451:string)  [unwired: 2 in, 2 out]
            n253 = Array Size(array=w444) -> (size(s)=w445:i32)
            n254 = local read "Gain error"() -> (w453:dbl[])
            n255 = Array Size(array=w443) -> (size(s)=w447:i32)
            n256 = local read "THD+N"() -> (w458:dbl[])
            n257 = Array Size(array=w437) -> (size(s)=w441:i32)
            n258 = call <vilib>:"DAQmx Unflatten Channel String.vi"("names in"=w451) -> ("names out"=w450:string[])  [unwired: 13 in, 1 out]
            n259 = Array Size(array=w438) -> (size(s)=w439:i32)
            n260 = local read "SFDR"() -> (w452:dbl[])
            n261 = local read "THD"() -> (w459:dbl[])
            n262 = local read "SNR"() -> (w454:dbl[])
            n263 = Divide(x=w447, y=w445) -> (x/y=w446:dbl)
            n264 = Divide(x=w439, y=w441) -> (x/y=w440:dbl)
            n265 = for {
              N: w445 -> [_]
              tunnel: w446 -> [w470]
              tunnel: [w471] -> w442 mode=indexing
              shift-right: [w472] -> _
              shift-left: w443 -> [w473]
              n266 = Delete From Array(array=w473, length=w470, index=0) -> (deleted portion=w471:dbl[], array with subset deleted=w472:dbl[])
            }
            n267 = for {
              tunnel: w459 -> [w515] mode=indexing
              tunnel: w458 -> [w514] mode=indexing
              tunnel: w457 -> [w513] mode=indexing
              tunnel: [w506] -> w434 mode=indexing
              tunnel: w456 -> [w505] mode=indexing
              tunnel: w455 -> [w504] mode=indexing
              tunnel: w454 -> [w503] mode=indexing
              tunnel: w453 -> [w501] mode=indexing
              tunnel: w452 -> [w500] mode=indexing
              tunnel: w450 -> [w495] mode=indexing
              w502 = "|   " ("initial string")
              n268 = Build Array(w505, w504) -> (w510:dbl[])
              n269 = Build Array(w503, w514, w515, w513) -> (w509:dbl[])
              n270 = for {
                tunnel: w510 -> [w520] mode=indexing
                tunnel: w502 -> [w521]
                tunnel: "%.3f" ("initial string") -> [w522]
                tunnel: [w523] -> w508 mode=indexing
                n271 = Format Into String(format string=w522, initial string=w521, w520) -> (resulting string=w523:string)  [unwired: 1 in, 1 out]
              }
              n272 = for {
                tunnel: w509 -> [w516] mode=indexing
                tunnel: w502 -> [w517]
                tunnel: "%5.1f" ("initial string") -> [w518]
                tunnel: [w519] -> w507 mode=indexing
                n273 = Format Into String(format string=w518, initial string=w517, w516) -> (resulting string=w519:string)  [unwired: 1 in, 1 out]
              }
              n274 = Format Into String(format string="%5.1f" ("initial string"), initial string=w502, w500) -> (resulting string=w498:string)  [unwired: 1 in, 1 out]
              n275 = Format Into String(format string="%5.3f" ("initial string"), initial string=w502, w501) -> (resulting string=w499:string)  [unwired: 1 in, 1 out]
              n276 = Concatenate Strings("Channel " ("string"), w495) -> (w494:string)
              n277 = Build Array (concatenate)(w494, w508, w507, w499, w498) -> (w506:string[])
            }
            "MeasTable" <- w434
            n278 = for {
              N: w441 -> [_]
              tunnel: w440 -> [w465]
              tunnel: [w466] -> w436 mode=indexing
              shift-right: [w467] -> _
              shift-left: w438 -> [w468]
              n279 = Delete From Array(array=w468, length=w465, index=0) -> (deleted portion=w466:dbl[], array with subset deleted=w467:dbl[])
            }
            n280 = local read "f0"() -> (w448:dbl[])
            n281 = for {
              tunnel: w442 -> [w491] mode=indexing
              tunnel: [w490] -> w449 mode=indexing
              tunnel: w448 -> [w489] mode=indexing
              tunnel: w444 -> [w488] mode=indexing
              n282 = Bundle(cluster=cluster{"x0":dbl, "dx":dbl, "magnitude":dbl[]} {"x0"=0.0, "dx"=0.0, "magnitude"=[]} ("FreqDomainGraph"), "x0"=w489, "dx"=w488, "magnitude"=w491) -> (w490:cluster{"x0":dbl, "dx":dbl, "magnitude":dbl[]})
            }
            n283 = for {
              tunnel: w437 -> [w463] mode=indexing
              tunnel: w436 -> [w462] mode=indexing
              tunnel: [w461] -> w435 mode=indexing
              n284 = Bundle By Name("dt"=w463, "Y"=w462) -> (w461:waveform(dbl))  [unwired: 1 in]
            }
            n285 = flat-sequence {
              tunnel: w449 -> [w475]
              tunnel: w435 -> [w474]
              tunnel: w432 -> [w478]
              tunnel: w429 -> [w477]
              tunnel: w427 -> [w476]
              frame #0 {
                "TimeDomainGraph" <- w474
                "FreqDomainGraph" <- w475
              }
              frame #1 {
                n286 = for {
                  tunnel: w478 -> [w479] mode=indexing
                  tunnel: w477 -> [w486]
                  tunnel: w476 -> [w485]
                  tunnel: w477 -> [w481]
                  tunnel: w476 -> [w480]
                  i -> [w483]
                  w482 = TRUE ("Legend:Plot Visibility Checkbox Visible")
                  w487 = TRUE ("Legend:Plot Visibility Checkbox Visible")
                  n287 = property on="FreqDomainGraph" class="WFGraph (strict)"("Active Plot"=w483, "PlotVisCheckbox"=w487, "LegAutosize"=w487, "LegNumRows"=w486, "LegScrollVis"=w485, "Plot.Plot Name"=w479) -> (error out=w484:errorcluster)  [unwired: 2 in, 1 out]
                  n288 = property on="TimeDomainGraph" class="WFGraph (strict)"(error in=w484, "Active Plot"=w483, "PlotVisCheckbox"=w482, "LegAutosize"=w482, "LegNumRows"=w481, "LegScrollVis"=w480, "Plot.Plot Name"=w479) -> ()  [unwired: 1 in, 2 out]
                }
              }
            }
            n289 = Index Array(array=w434, index (col)=0 ("disabled index (col)")) -> (element=w432:string[])  [unwired: 1 in]
            n290 = Array Size(array=w432) -> (size(s)=w431:i32)
            n291 = Less Or Equal?(x=w431, y=w430) -> (x <= y?=w428:bool)
            n292 = Not(x=w428) -> (.not. x?=w427:bool)
            n293 = Select(t=w431, s=w428, f=w430) -> (s? t:f=w429:i32)
          }
          frame "Exit" {
            # "This case is triggered to close the User Interface from framework"
            n294 = Flush Queue(queue=w528, error in (no error)=w530) -> (queue out=w527:refnum<queue>, error out=w526:errorcluster)  [unwired: 1 out]
            n295 = Release Queue(queue=w527, force destroy? (F)=TRUE, error in (no error)=w526) -> (error out=w525:errorcluster)  [unwired: 2 out]
          }
          frame "Handle Error" {
          }
        }
      }
    }
  }
